vi "testprop timing source.vi"() -> ()   [LabVIEW 2013, in "TBM Tests.lvlib"]
uses:
  TBM Tests.lvlib
  module configuration/TBM module configuration.lvclass
  module configuration/timing source.ctl
panel:
  out "no error":errorcluster
  out "source=none":bool
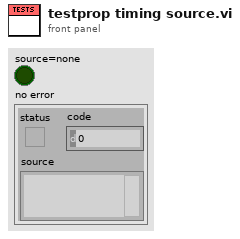
[diagram p1: front panel]
types:
  T1 = typedef "TBM module configuration.lvclass/timing source.ctl" = enum16{"None", "Custom Timing Source", "1 kHz Clock", "1 MHz Clock", "Synchronize to Scan Engine"}
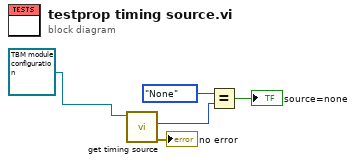
[diagram p0: block diagram]
diagram:
  n1 = call-dynamic "get timing source.vi"("module configuration in"=refnum<class "TBM module configuration.lvclass"> refnum ("module configuration")) -> ("error out"=→"no error":errorcluster, "timing source enum"=w4:T1)  [unwired: 8 in, 1 out]
  n2 = Equal?(x=timing_source."None", y=w4) -> (x = y?=→"source=none":bool)
